vi "HornScan_BelowMax_30KHZ_Test.vi"() -> ()   [LabVIEW 2017]
panel:
  out "HORN scan progress":string
  out "String":string
  out "Error Out":errorcluster={"status"=FALSE, "code"=-1, "source"=""}
  out "HORN SCAN Test Result":picture
  out "Response time graph":cluster{dbl, u32}[](graph)=[{3630033366.1128, 18791}]
  # "Range of HORN SCAN Recipe parameter"
  # "Range of HORN SCAN recipe parameters\nStart Frequency=19450 to 20450(20Hz); \n                              29400 to 36000(30Hz); \n                              39100 to 40700(40Hz); \nStop Frequency=19450 to 20450Hz\nFrequency Step=1 to 100Hz\nTime Delay=0.01 to 0.1s\nMax Amplitude=1 to 100%\nMax Current=1 to 100%\nSetDigitalTuneWithHornScan=0 or 1"
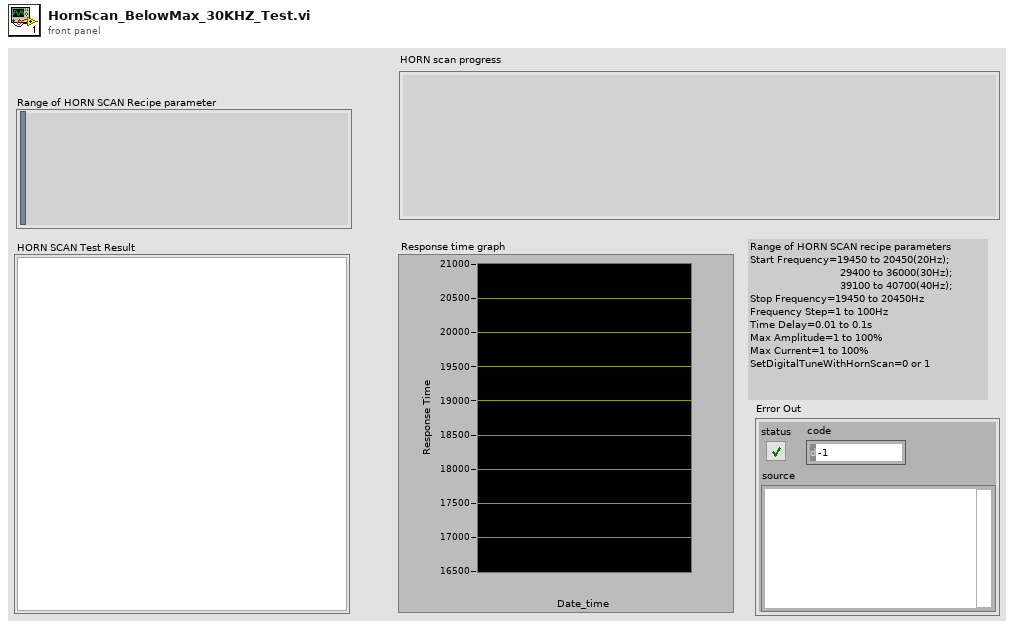
[diagram p1: front panel]
types:
  T1 = enum16{"open", "replace", "create", "open or create", "replace or create", "replace or create with confirmation"}
  T2 = cluster{"[0]":string, "[1]":string, "[2]":string, "[3]":string, "[4]":string, "[5]":string, "[6]":string, "[7]":string, "[8]":string}
  T3 = cluster{"Iterations":u64, "DelayBetweenIterations":u32, "Timeout":u32, "MessageID":u32, "MessageLength":u32, "ResponseID":i32, "Start Frequency":u32, "Stop Frequency":u32, "Frequency Step":u16, "Time Delay":u16, "Max Amplitude":u16, "Max Current":u16, "SetDigitalTuneWithHornScan":u16, "Timestamp":string, "TestSuite":string, "ReportPath":path, "FWVersionPath":path}
  T4 = cluster{"Socket_IP_Address":string, "Socket_Port_Number":u16, "Global_ReportPath":path}
  T5 = typedef "imagedata.ctl" = cluster{"image type":i32, "image depth":i32, "image":u8[], "mask":u8[], "colors":u32[], "Rectangle":cluster{"left":i16, "top":i16, "right":i16, "bottom":i16}}
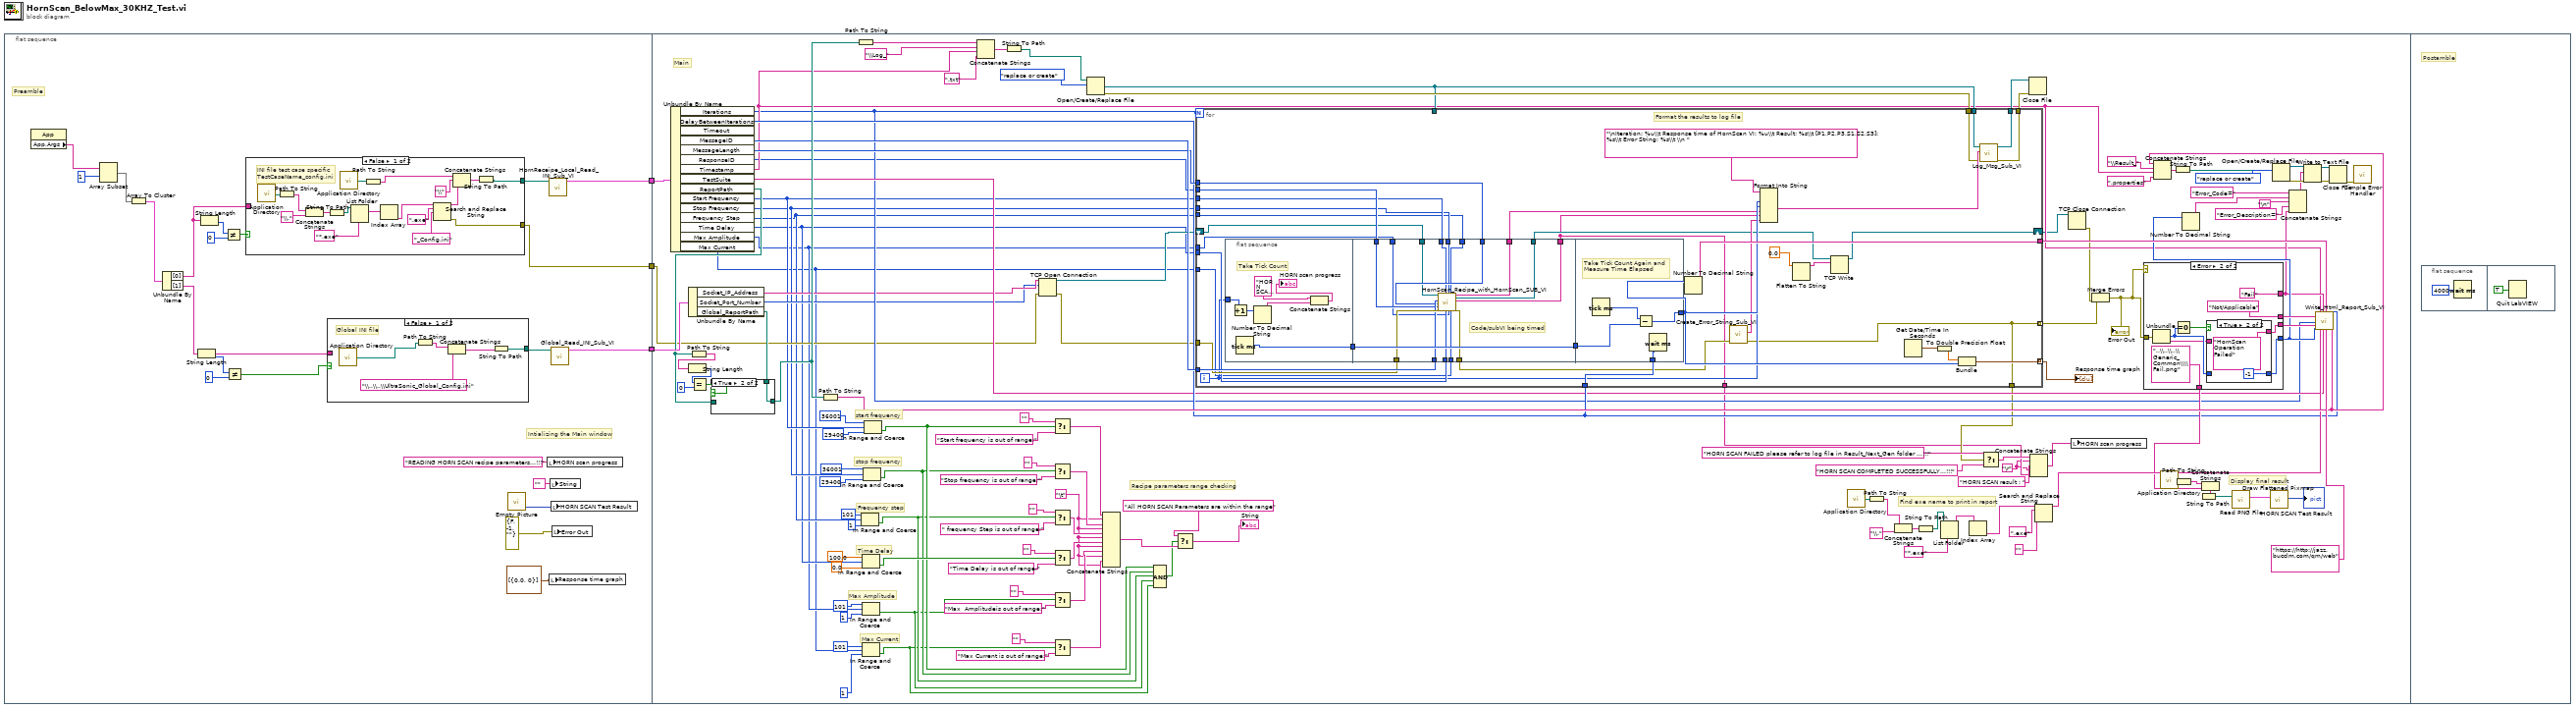
[diagram p0: block diagram]
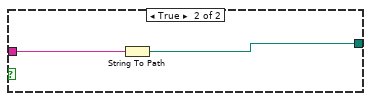
[diagram p2: hidden frame]
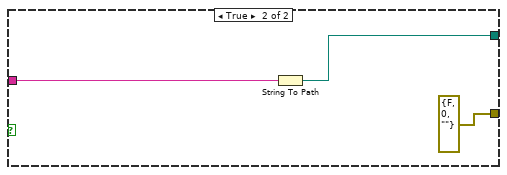
[diagram p3: hidden frame]
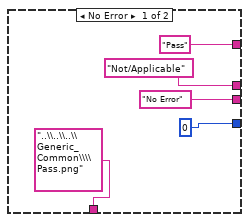
[diagram p5: hidden frame]
diagram:
  n1 = flat-sequence {
    tunnel: [w11] -> w3
    tunnel: [w10] -> w2
    tunnel: [w9] -> w1
    tunnel: w3 -> [w112]
    tunnel: w2 -> [w126]
    tunnel: w1 -> [w117]
    frame #0 {
      # "Intializing the Main window"
      # "Preamble"
      n2 = property class="App"() -> ("App.Args"=w13:string[])  [unwired: 2 in, 2 out]
      n3 = Array Subset "Array Subset"(array=w13, index=1) -> (w14:string[])  [unwired: 1 in]
      n4 = Array To Cluster(array=w14) -> (cluster=w15:T2)
      n5 = Unbundle By Name "Unbundle By Name"(w15) -> ("[0]"=w19:string, "[1]"=w22:string)
      n6 = String Length(string=w22) -> (length=w23:i32)
      n7 = String Length(string=w19) -> (length=w16:i32)
      n8 = Not Equal?(x=w16, y=0) -> (x != y?=w18:bool)
      n9 = Not Equal?(x=w23, y=0) -> (x != y?=w21:bool)
      n10 = case shown="False" w18 {
        tunnel: w19 -> [_ w52]
        tunnel: [w34 w51] -> w24
        tunnel: [w33 errorcluster {"status"=FALSE, "code"=0, "source"=""} ("error out")] -> w11
        frame False {
          # "INI file test case specific\nTestCaseName_config.ini"
          n11 = call <vilib>:"Application Directory.vi"() -> ("Application Directory"=w40:path)
          n12 = Path To String(path=w40) -> (string=w39:string)
          n13 = Concatenate Strings(w39, "\\." ("string")) -> (w37:string)
          n14 = String To Path(string=w37) -> (path=w42:path)
          n15 = call <vilib>:"Application Directory.vi"() -> ("Application Directory"=w49:path)
          n16 = List Folder(path=w42, pattern="*.exe") -> (filenames=w36:string[])  [unwired: 2 in, 3 out]
          n17 = Path To String(path=w49) -> (string=w44:string)
          n18 = Index Array(array=w36) -> (element=w35:string)  [unwired: 1 in]
          n19 = Search and Replace String(input string=w35, search string=".exe", replace string="_Config.ini" ("replace string (\"\")")) -> (result string=w46:string, error out=w33:errorcluster)  [unwired: 5 in, 2 out]
          n20 = Concatenate Strings(w44, "\\" ("string"), w46) -> (w43:string)
          n21 = String To Path(string=w43) -> (path=w34:path)
        }
        frame True {
          n22 = String To Path(string=w52) -> (path=w51:path)
        }
      }
      n23 = case shown="False" w21 {
        tunnel: [w27 w32] -> w25
        tunnel: w22 -> [_ w31]
        frame False {
          # "Global INI file"
          n24 = call <vilib>:"Application Directory.vi"() -> ("Application Directory"=w26:path)
          n25 = Path To String(path=w26) -> (string=w30:string)
          n26 = Concatenate Strings(w30, "\\..\\..\\UltraSonic_Global_Config.ini" ("string")) -> (w28:string)
          n27 = String To Path(string=w28) -> (path=w27:path)
        }
        frame True {
          n28 = String To Path(string=w31) -> (path=w32:path)
        }
      }
      n29 = call "Empty Picture"() -> ("empty picture"=w5:picture)
      n30 = local write "HORN scan progress"("READING HORN SCAN recipe parameters...!!!" ("HORN scan progress")) -> ()
      n31 = call "HornReceipe_Local_Read_INI_Sub_VI.vi"("Config File Path"=w24) -> ("output cluster"=w9:T3)  [unwired: 10 in]
      n32 = local write "Response time graph"(cluster{dbl, u32}[] [{0.0, 0}] ("Response time graph")) -> ()
      n33 = local write "String"("" ("String")) -> ()
      n34 = call "Global_Read_INI_Sub_VI.vi"("Config File Path"=w25) -> ("output cluster"=w10:T4)  [unwired: 14 in]
      n35 = local write "HORN SCAN Test Result"(w5) -> ()
      n36 = local write "Error Out"(errorcluster {"status"=FALSE, "code"=-1, "source"=""} ("error out")) -> ()
    }
    frame #1 {
      w53 = "\r"
      w70 = "\t"
      # "Recipe parameters range checking"
      # "Max Current"
      # "Max Amplitude"
      # "Time Delay"
      # "Frequency step"
      # "stop frequency"
      # "start frequency"
      # "Display final result"
      # "Find exe name to print in report"
      # "Main"
      n37 = Unbundle By Name(w117) -> ("Iterations"=w118:u64, "DelayBetweenIterations"=w122:u32, "MessageID"=w124:u32, "MessageLength"=w123:u32, "ResponseID"=w115:i32, "Timestamp"=w120:string, "TestSuite"=w119:string, "ReportPath"=w116:path, "Start Frequency"=w107:u32, "Stop Frequency"=w106:u32, "Frequency Step"=w105:u16, "Time Delay"=w104:u16, "Max Amplitude"=w103:u16, "Max Current"=w102:u16)  [unwired: 1 out]
      n38 = Unbundle By Name(w126) -> ("Socket_IP_Address"=w114:string, "Socket_Port_Number"=w113:u16, "Global_ReportPath"=w125:path)
      n39 = Path To String(path=w116) -> (string=w173:string)
      n40 = String Length(string=w173) -> (length=w172:i32)
      n41 = Equal?(x=w172, y=0) -> (x = y?=w170:bool)
      n42 = case shown="True" w170 {
        tunnel: w125 -> [_ w185]
        tunnel: [w184 w185] -> w169
        tunnel: w116 -> [w184 _]
        frame False {
        }
        frame True {
        }
      }
      n43 = Path To String(path=w169) -> (string=w146:string)
      n44 = Path To String(path=w169) -> (string=w175:string)
      n45 = In Range and Coerce(upper limit=i16 101, x=w105, lower limit=i16 1) -> (In Range?=w59:bool)  [unwired: 1 out]
      n46 = In Range and Coerce(upper limit=100.0, x=w104, lower limit=0.0) -> (In Range?=w82:bool)  [unwired: 1 out]
      n47 = In Range and Coerce(upper limit=i16 101, x=w103, lower limit=i16 1) -> (In Range?=w58:bool)  [unwired: 1 out]
      n48 = In Range and Coerce(upper limit=i16 101, x=w102, lower limit=i16 1) -> (In Range?=w57:bool)  [unwired: 1 out]
      n49 = In Range and Coerce(upper limit=36001, x=w106, lower limit=29400) -> (In Range?=w60:bool)  [unwired: 1 out]
      n50 = In Range and Coerce(upper limit=36001, x=w107, lower limit=29400) -> (In Range?=w61:bool)  [unwired: 1 out]
      n51 = Concatenate Strings(w175, "\\Log_" ("string"), w120, ".txt" ("string")) -> (w178:string)
      n52 = String To Path(string=w178) -> (path=w177:path)
      n53 = TCP Open Connection(address=w114, remote port or service name=w113, error in (no error)=w112) -> (connection ID=w108:refnum<k5>, error out=w111:errorcluster)  [unwired: 2 in]
      n54 = Select(t="", s=w61, f="Start frequency is out of range;") -> (s? t:f=w76:string)
      n55 = Select(t="", s=w60, f="Stop frequency is out of range;") -> (s? t:f=w75:string)
      n56 = Select(t="", s=w59, f=" frequency Step is out of range;") -> (s? t:f=w74:string)
      n57 = Select(t="", s=w82, f="Time Delay is out of range;") -> (s? t:f=w73:string)
      n58 = Select(t="", s=w58, f="Max  Amplitudeis out of range;") -> (s? t:f=w72:string)
      n59 = Select(t="", s=w57, f="Max Current is out of range;") -> (s? t:f=w71:string)
      n60 = Open/Create/Replace File(file path (use dialog)=w177, operation (0:open)=T1."replace or create") -> (refnum out=w147:refnum<file>, error out=w150:errorcluster)  [unwired: 1 in, 4 out]
      n61 = Concatenate Strings(w76, w70, w75, w70, w74, w70, w73, w70, w72, w70, w71, w70) -> (w62:string)
      n62 = Compound Arithmetic op=AND(w61, w60, w59, w58, w57) -> (w56:bool)
      n63 = Select(t="All HORN SCAN Parameters are within the range" ("f"), s=w56, f=w62) -> (s? t:f=→"String":string)
      n64 = for {
        N: w118 -> [_]
        tunnel: [w218] -> w181
        tunnel: w147 -> [w212]
        tunnel: [w211] -> w149
        tunnel: [w209] -> w148
        tunnel: [w214] -> w179 mode=indexing
        tunnel: w150 -> [w210]
        tunnel: w147 -> [_]
        tunnel: [w191] -> w145 mode=indexing
        tunnel: w124 -> [w207]
        tunnel: w123 -> [w206]
        tunnel: w115 -> [w204]
        tunnel: w122 -> [w205]
        tunnel: w111 -> [w203]
        tunnel: w107 -> [w200]
        tunnel: w106 -> [w199]
        tunnel: w105 -> [w198]
        tunnel: w104 -> [w197]
        tunnel: w103 -> [w196]
        tunnel: w102 -> [w195]
        shift-right: [w189] -> w109
        shift-left: w108 -> [w194]
        tunnel: [w186] -> w54
        tunnel: [w191] -> w66
        i -> [w193]
        # "Format the results to log file"
        n65 = flat-sequence {
          tunnel: [w226] -> w220
          tunnel: w193 -> [w222]
          tunnel: [w242] -> w219
          tunnel: w220 -> [w242]
          tunnel: w207 -> [w237]
          tunnel: w206 -> [w236]
          tunnel: w204 -> [w235]
          tunnel: [w240] -> w192
          tunnel: w203 -> [w238]
          tunnel: [w241] -> w186
          tunnel: [w239] -> w201
          tunnel: w200 -> [w234]
          tunnel: w199 -> [w233]
          tunnel: w198 -> [w232]
          tunnel: w197 -> [w231]
          tunnel: w196 -> [w230]
          tunnel: w195 -> [w229]
          tunnel: w194 -> [w228]
          tunnel: [w227] -> w190
          tunnel: w219 -> [w246]
          tunnel: [w244] -> w208
          tunnel: w205 -> [w243]
          frame #0 {
            # "Take Tick Count"
            n66 = Increment(x=w222) -> (x+1=w221:i32)
            n67 = Tick Count (ms)() -> (millisecond timer value=w226:u32)
            n68 = Number To Decimal String(number=w221) -> (decimal integer string=w224:string)  [unwired: 1 in]
            n69 = Concatenate Strings("HORN SCAN INPROGRESS....!!!\nIteration - ", w224) -> (→"HORN scan progress":string)
          }
          frame #1 {
            # "Code/subVI being timed"
            n70 = call "HornScan_Recipe_with_HornScan_SUB_VI.vi"("connection ID"=w228, "Receipe Msg ID"=w237, "Receipe Message length"=w236, "Response ID"=w235, "error in (no error)"=w238, "Start Frequency"=w234, "Time Delay"=w231, "Stop Frequency"=w233, "Max Amplitude"=w230, "Frequency Step"=w232, "Max Current"=w229) -> ("Pass"=w240:string, "connection ID_out"=w227:refnum<k5>, "Resonant Frequencies"=w241:string, "error out"=w239:errorcluster)  [unwired: 5 in]
          }
          frame #2 {
            # "Take Tick Count Again and Measure Time Elapsed"
            n71 = Tick Count (ms)() -> (millisecond timer value=w245:u32)
            n72 = Subtract(x=w245, y=w246) -> (x-y=w244:u32)
            n73 = Wait (ms)(milliseconds to wait=w243) -> ()  [unwired: 1 out]
          }
        }
        n74 = Number To Decimal String(number=w208) -> (decimal integer string=w218:string)  [unwired: 1 in]
        n75 = call "Create_Error_String_Sub_VI.vi"("error in"=w201) -> ("error out"=w191:errorcluster, "Error String"=w202:string)  [unwired: 9 in]
        n76 = Format Into String(format string="\nIteration: %u\\t Response time of HornScan VI: %u\\t Result: %s\\t [P1,P2,P3,S1,S2,S3]: %s\\t Error String: %s\\t \\n ", w193, w208, w192, w186, w202) -> (resulting string=w213:string)  [unwired: 2 in, 1 out]
        n77 = Flatten To String(anything=0.0) -> (data string=w188:string)  [unwired: 3 in, 2 out]
        n78 = TCP Write(connection ID=w190, data in=w188) -> (connection ID out=w189:refnum<k5>)  [unwired: 2 in, 2 out]
        n79 = Get Date/Time In Seconds() -> (seconds since 1Jan1904=w215:timestamp)
        n80 = To Double Precision Float(number=w215) -> (double precision float=w216:dbl)
        n81 = Bundle "Bundle"(w216, w208) -> (w214:cluster{dbl, u32})  [unwired: 1 in]
        n82 = call "Log_Msg_Sub_VI.vi"("error in (no error)"=w210, "String"=w213, "Byte Stream File in"=w212) -> ("error out"=w209:errorcluster, "Byte Stream File out"=w211:refnum<file>)  [unwired: 7 in]
      }
      "Response time graph" <- w179
      n83 = call <vilib>:"Application Directory.vi"() -> ("Application Directory"=w142:path)
      n84 = Path To String(path=w142) -> (string=w141:string)
      n85 = Concatenate Strings(w141, "\\." ("string")) -> (w139:string)
      n86 = String To Path(string=w139) -> (path=w144:path)
      n87 = List Folder(path=w144, pattern="*.exe") -> (filenames=w138:string[])  [unwired: 2 in, 3 out]
      n88 = Index Array(array=w138) -> (element=w134:string)  [unwired: 1 in]
      n89 = Select(t="HORN SCAN FAILED please refer to log file in Result_Next_Gen folder ...!!!", s=w66, f="HORN SCAN COMPLETED SUCCESSFULLY...!!!") -> (s? t:f=w65:string)
      n90 = Close File(refnum=w149, error in=w148) -> ()  [unwired: 2 out]
      n91 = Concatenate Strings(w65, w53, "HORN SCAN result : " ("string"), w53, w54) -> (w67:string)
      n92 = Search and Replace String(input string=w134, search string=".exe", replace string="" ("replace string (\"\")")) -> (result string=w137:string)  [unwired: 5 in, 3 out]
      n93 = TCP Close Connection(connection ID=w109) -> (error out=w110:errorcluster)  [unwired: 2 in, 1 out]
      n94 = local write "HORN scan progress"(w67) -> ()
      n95 = Merge Errors "Merge Errors"(w145, w110) -> (w121:errorcluster)
      "Error Out" <- w121
      n96 = case shown="Error" w121 {
        tunnel: ["Pass" "Fail"] -> w151
        tunnel: w121 -> [_ w258]
        tunnel: [0 ("code") w254] -> w155
        tunnel: ["No Error" ("source") w255] -> w183
        tunnel: ["Not/Applicable" "Not/Applicable"] -> w182
        tunnel: ["..\\..\\..\\Generic_Common\\\\Pass.png" ("string") "..\\..\\..\\Generic_Common\\\\Fail.png" ("string")] -> w127
        frame No Error {
        }
        frame Error {
          n97 = Unbundle(w258) -> ("code"=w256:i32, "source"=w252:string)  [unwired: 1 out]
          n98 = Equal To 0?(x=w256) -> (x = 0?=w253:bool)
          n99 = case shown="True" w253 {
            tunnel: [w262 -1 ("code")] -> w254
            tunnel: [w261 "HornScan Operation Failed" ("source")] -> w255
            tunnel: w256 -> [w262 _]
            tunnel: w252 -> [w261 _]
            frame False {
            }
            frame True {
            }
          }
        }
      }
      n100 = Concatenate Strings(w146, "\\Result_" ("string"), w120, ".properties" ("string")) -> (w167:string)
      n101 = call <vilib>:"Application Directory.vi"() -> ("Application Directory"=w128:path)
      n102 = String To Path(string=w167) -> (path=w159:path)
      n103 = Path To String(path=w128) -> (string=w129:string)
      n104 = Number To Decimal String(number=w155) -> (decimal integer string=w154:string)  [unwired: 1 in]
      n105 = Concatenate Strings(w129, w127) -> (w130:string)
      n106 = String To Path(string=w130) -> (path=w133:path)
      n107 = call <vilib>:"Read PNG File.vi"("path to PNG file"=w133) -> ("image data"=w131:T5)  [unwired: 8 in, 2 out]
      n108 = call <vilib>:"Draw Flattened Pixmap.vi"("image data"=w131) -> ("new picture"=→"HORN SCAN Test Result":picture)  [unwired: 8 in]
      n109 = Open/Create/Replace File(file path (use dialog)=w159, operation (0:open)=T1."replace or create") -> (refnum out=w158:refnum<file>, error out=w163:errorcluster)  [unwired: 4 in, 1 out]
      n110 = Concatenate Strings("Error_Code=" ("string"), w154, "\n", "Error_Description=" ("string"), w151) -> (w157:string)
      n111 = Write to Text File(file (use dialog)=w158, text=w157, error in=w163) -> (refnum out=w162:refnum<file>, error out=w161:errorcluster)  [unwired: 1 in, 1 out]
      n112 = call "Write_Html_Report_Sub_VI.vi"("ReprtPath"=w146, "Remarks"=w182, "Iterations"=w118, "Error Description"=w183, "Timestamp"=w120, "TestCase"=w137, "Verdict"=w151, "TestSuite"=w119, "Time taken to execute  test in msec"=w181, "JazzDashboardLink"="https://http://jazz.bucclm.com/qm/web" ("TestSuite"), "Delay Between Iterations"=w122, "Error Code"=w155) -> ()  [unwired: 8 in]
      n113 = Close File(refnum=w162, error in=w161) -> (error out=w160:errorcluster)  [unwired: 1 out]
      n114 = call <vilib>:"Simple Error Handler.vi"("error in (no error)"=w160) -> ()  [unwired: 4 in, 5 out]
    }
    frame #2 {
      # "Postamble"
      n115 = flat-sequence {
        frame #0 {
          n116 = Wait (ms)(milliseconds to wait=u32 4000) -> ()  [unwired: 1 out]
        }
        frame #1 {
          n117 = Quit LabVIEW(quit? (T)=TRUE) -> ()
        }
      }
    }
  }
